vi "Read MT Name.vi"(11 "Message Interface in":refnum<class "Message Interface.lvclass">) -> (2 "MT Name":string, 3 "Message Interface out":refnum<class "Message Interface.lvclass">)   [LabVIEW 2016, in "Stream Mediator.lvlib" / "Message Interface.lvclass"]
doc: "--\nCopyright © 2017 Composed SystemsI All rights reserved.\n\nAuthor: Jon McBee <jon.mcbee@composed.io>\n\nThis library is provided \"AS IS\" ,WITHOUT WARRANTIES OR\nCONDITIONS OF ANY KIND, either express or implied.\n\nComposed Systems -- composed.io\n\nStream 0.0.1.1\nJon McBee - Composed Systems\nCopyright (c) 2017, Composed Systems"
uses:
  <userlib>/Composed Systems/Stream/Mediator/Classes/Message Interface/Message Interface.lvclass
  <userlib>/Composed Systems/Stream/Mediator/Classes/Message Interface/Message Interface.lvclass/Message Interface.ctl
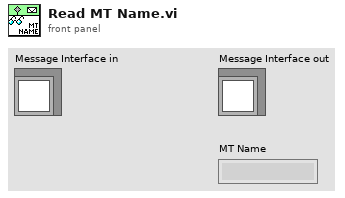
[diagram p1: front panel]
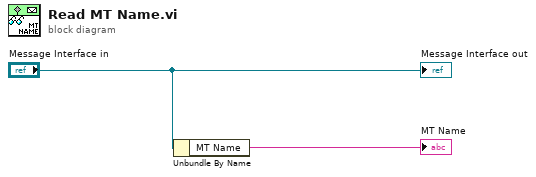
[diagram p0: block diagram]
diagram:
  n1 = Unbundle By Name("Message Interface in") -> ("MT Name"=→"MT Name":string)
  "Message Interface out" <- "Message Interface in"
